vi "PH_IEEE1394Camera.ProcCases.vi"(0 "i ref in":refnum<vi>, 1 "selector":string, 2 "data":T1, 3 "call cluster":T2={"Object"="", "Selector"="", "CallType"=enum."synchronous", "Async Object"="", "Async Selector"="", "Data Descriptor"="", "Data"=[], "Error #"=0, "Expire"=0}, 5 "error in":errorcluster) -> (14 "i ref out":refnum<vi>, 17 "answer cluster":T2={"Object"="", "Selector"="", "CallType"=enum."synchronous", "Async Object"="", "Async Selector"="", "Data Descriptor"="", "Data"=[], "Error #"=0, "Expire"=0}, 19 "error out":errorcluster)   [LabVIEW 2014, in "PH_IEEE1394Camera.lvlib"]
doc: "This method is called by a process from within the default case in the event loop. The methods of a class that are linked to events will be called from THIS method. Add your code here."
uses:
  PH_IEEE1394Camera.lvlib
  CS_Core/CSSystem/CoreDefs/CoreDefs.call_type.ctl
  CS_Core/BaseProcess/BaseProcess.descriptor string definition.ctl
  CS_Core/CSSystem/CoreDefs/CoreDefs.rawDataType.ctl
  CS_Core/CSSystem/CoreLib/CoreLib.string 2 byte array.vi
  CS_Core/CSSystem/CoreLib/CoreLib.byte array 2 int.vi
  CS_Core/CSSystem/CoreLib/CoreLib.byte array 2 double.vi
  CS_Core/CSSystem/CoreLib/CoreLib.byte array 2 short.vi
  CS_Core/CSSystem/CoreLib/CoreLib.byte array 2 string.vi
  CS_Core/CSSystem/CoreLib/CoreLib.lvlib
  CS_Core/BaseProcess/BaseProcess.lvlib
  CS_Core/CAEObj/CAEObj.lvlib
  PH_Basics/PH_PSDBWriter/PH_PSDBWriter.lvlib
  PH_Basics/PH_Cam_BaseClass/PH_Cam_BaseClass.lvlib
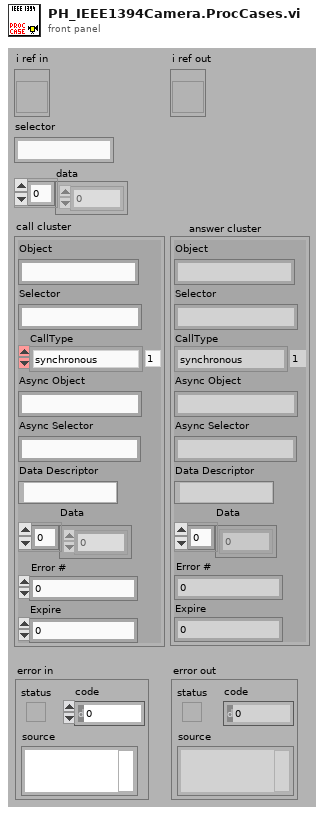
[diagram p1: front panel]
types:
  T1 = typedef "CoreDefs.rawDataType.ctl" = i8[]
  T2 = typedef "CoreDefs.call_type.ctl" = cluster{"Object":string, "Selector":string, "CallType":enum16{"simple", "synchronous", "asynchronous"}, "Async Object":string, "Async Selector":string, "Data Descriptor":T3, "Data":T1, "Error #":i32, "Expire":u32}
  T3 = typedef "BaseProcess.lvlib/BaseProcess.descriptor string definition.ctl" = string
  T4 = typedef "PH_PSDBWriter.lvlib/PH_PSDBWriter.PHELIX-Subsystems.ctl" = i32
  T5 = typedef "PH_IEEE1394Camera.lvlib/PH_IEEE1394Camera.i attribute.ctl" = cluster{"Gui Refs":cluster{"Brightness":refnum<vi>, "Shutter":refnum<vi>, "Gain":refnum<vi>, "Center of Gravity":refnum<vi>, "Supported Video Modes":refnum<vi>, "Trigger Polarity":refnum<vi>, "Trigger Mode":refnum<vi>, "Trigger Timeout":refnum<vi>, "Bit Depth":refnum<vi>, "Video Mode":refnum<vi>, "Top":refnum<vi>, "Bottom":refnum<vi>, "Left":refnum<vi>, "Right":refnum<vi>, "Set ROI to Maximum":refnum<vi>, "Camera Details":refnum<vi>, "Current Cam Attributes":refnum<vi>, "Attribute to set":refnum<vi>, "Num Value":refnum<vi>, "String Value":refnum<vi>, "Bool Value":refnum<vi>, "Set Cam Attribute":refnum<vi>}, "Cam":cluster{"IMAQ1394 Session":T6, "Camera Details":T7}, "Current Attributes":T8[], "Supported Video Modes ":cluster{"Video Mode":u32, "Video Mode Name":string}[], "Wanted Attributes":cluster{"Name":string, "Num Value":dbl, "String Value":string, "Boolean Value":bool}[], "Cam Attributes":T10}
  T6 = typedef "IMAQdx.ctl" = refnum<k21>
  T7 = typedef "PH_IEEE1394Camera.lvlib/PH_IEEE1394Camera.Cam Details.ctl" = cluster{"Model":string, "Serial Number":dbl, "Cam name (Machinery)":string, "Bus Type":string}
  T8 = typedef "PH_IEEE1394Camera.lvlib/PH_IEEE1394Camera.Cam Attribute.ctl" = cluster{"Information":cluster{"Type":T9, "Readable":bool, "Writable":bool, "Name":string}, "Num Value":dbl, "String Value":string, "Maximum":dbl, "Minimum":dbl, "Units":string, "Description":string, "EnumStrings[]":string[], "EnumValues[]":u32[], "Boolean Value":bool}
  T9 = typedef "NI_Vision_Acquisition_Software.lvlib/IMAQdx Attribute Type.ctl" = enum32{"U32", "I64", "DBL", "String", "Enum", "Bool", "Command"}
  T10 = typedef "PH_IEEE1394Camera.lvlib/PH_IEEE1394Camera.Relevant Cam Attributes.ctl" = cluster{"Video Mode":cluster{"Name":string, "Index":i32}, "Brightness":cluster{"Name":string, "Index":i32}, "Gain":cluster{"Name":string, "Index":i32}, "Shutter":cluster{"Name":string, "Index":i32}, "Trigger Pol":cluster{"Name":string, "Index":i32}, "Trigger Mode":cluster{"Name":string, "Index":i32}, "Timeout":cluster{"Name":string, "Index":i32}, "Bit Depth":cluster{"Name":string, "Index":i32}, "Pixel Bits":cluster{"Name":string, "Index":i32}, "Pixel Bytes":cluster{"Name":string, "Index":i32}, "Left":cluster{"Name":string, "Index":i32}, "Right":cluster{"Name":string, "Index":i32}, "Top":cluster{"Name":string, "Index":i32}, "Bottom":cluster{"Name":string, "Index":i32}}
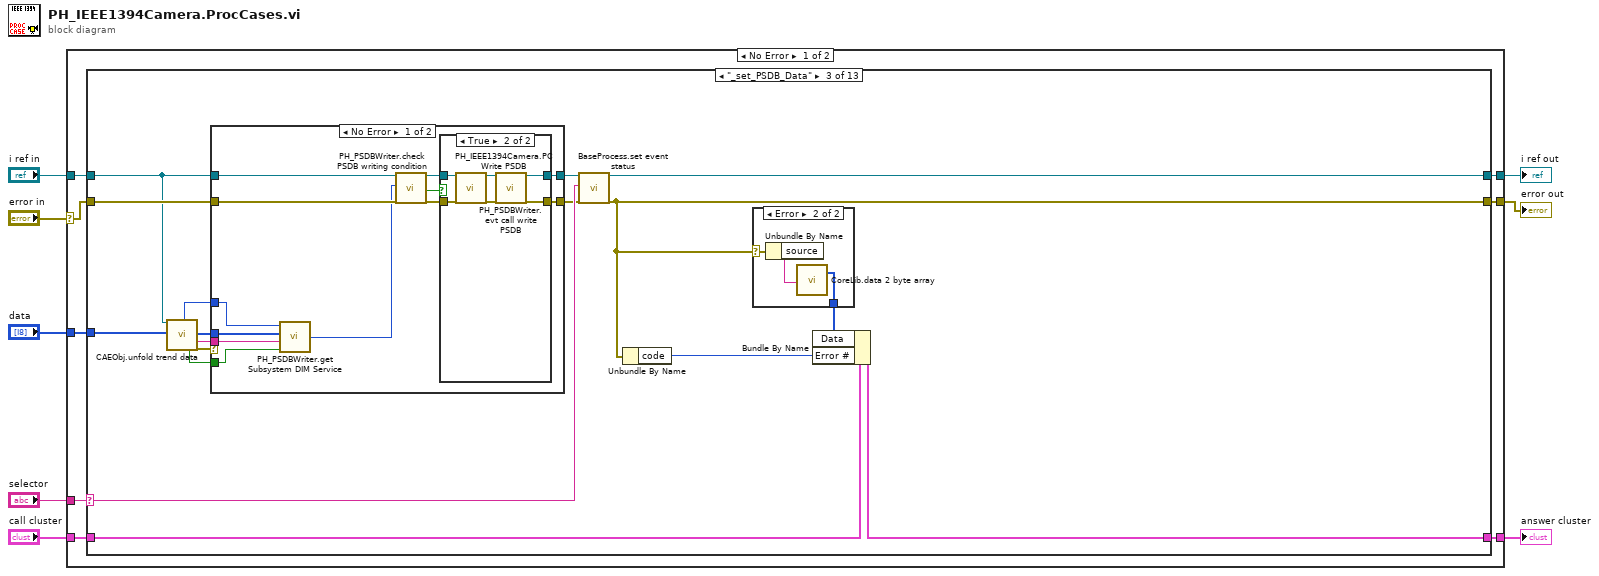
[diagram p0: block diagram]
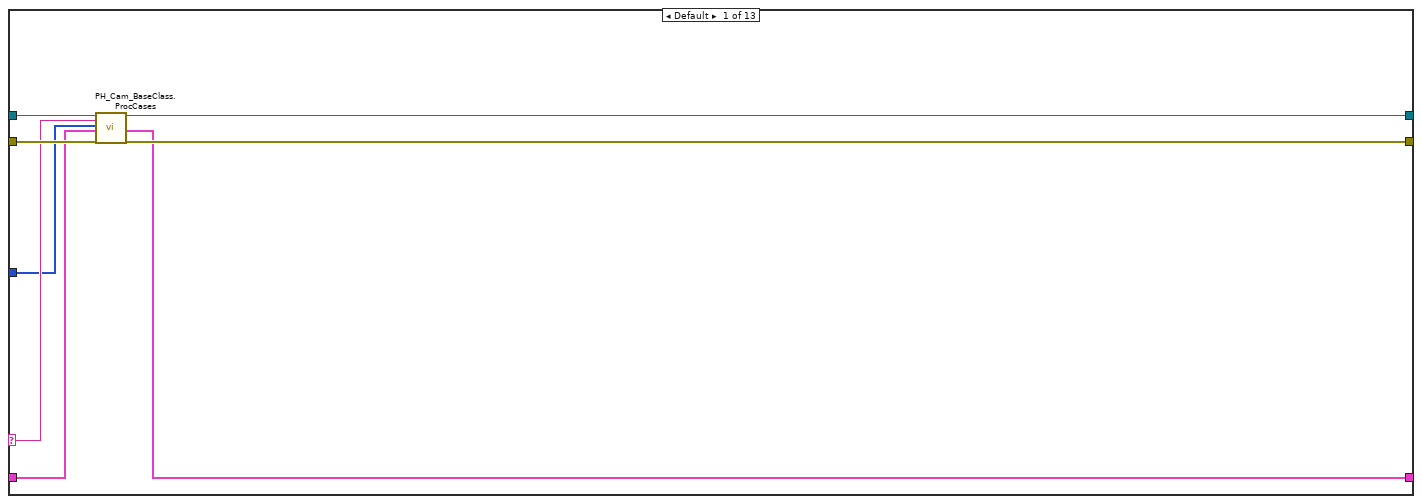
[diagram p2: hidden frame]
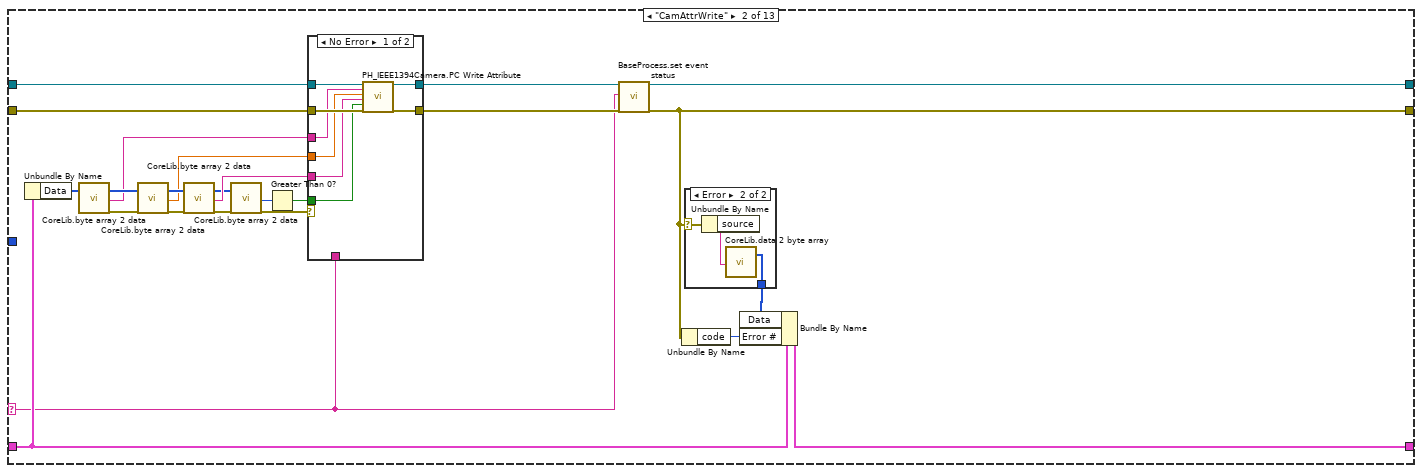
[diagram p3: hidden frame]
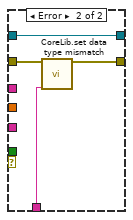
[diagram p5: hidden frame]
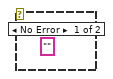
[diagram p8: hidden frame]
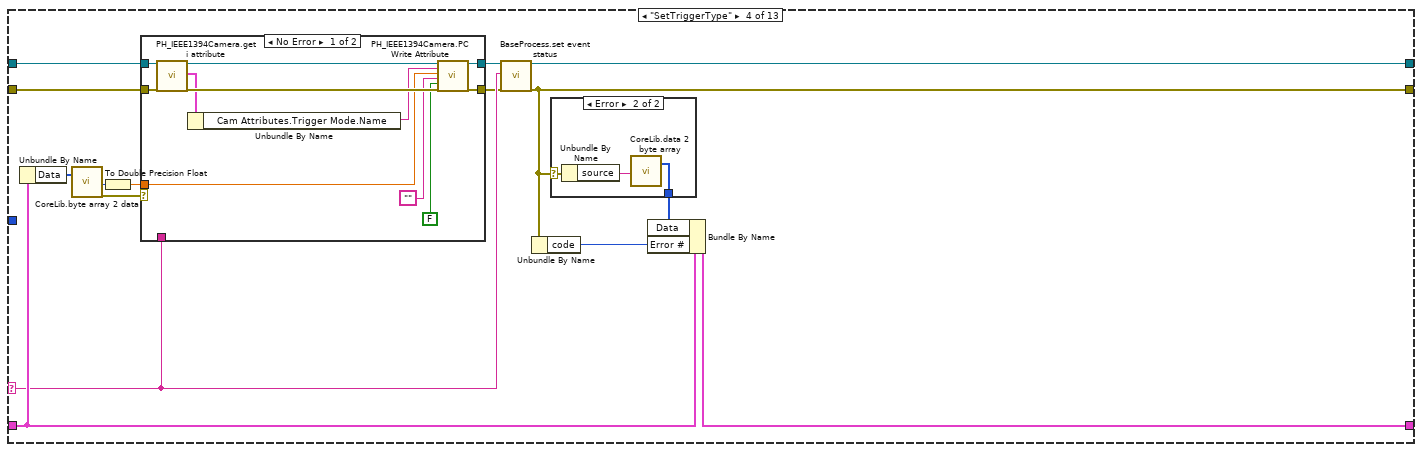
[diagram p9: hidden frame]
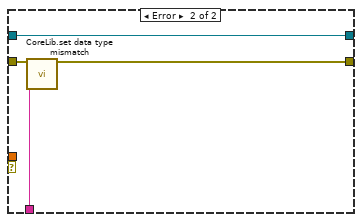
[diagram p10: hidden frame]
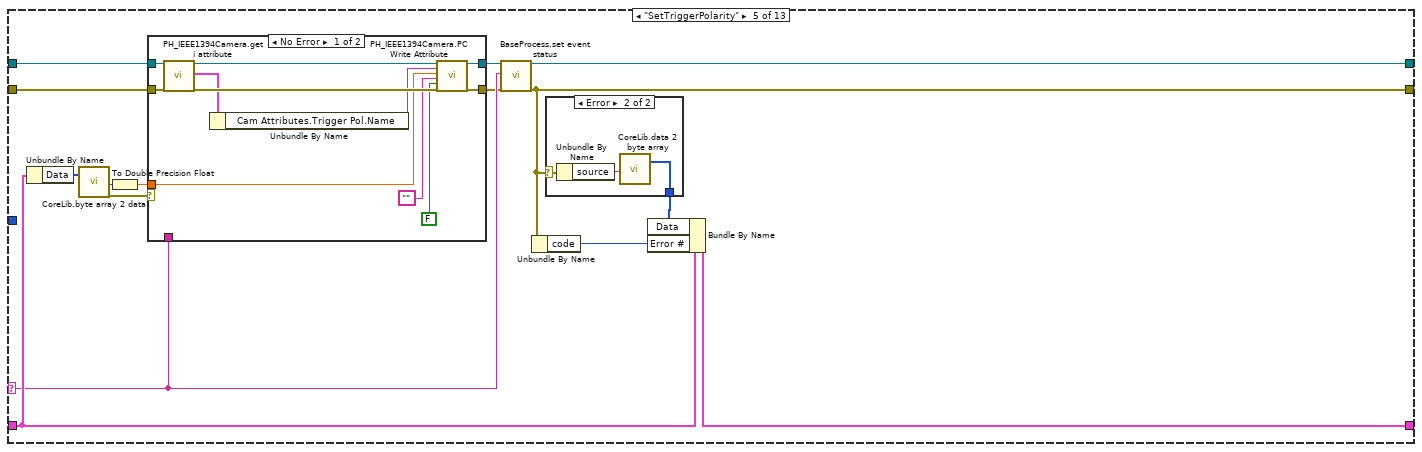
[diagram p12: hidden frame]
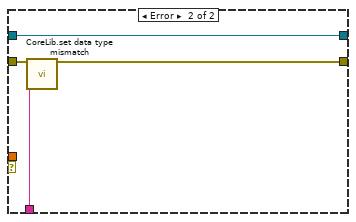
[diagram p13: hidden frame]
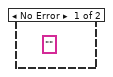
[diagram p14: hidden frame]
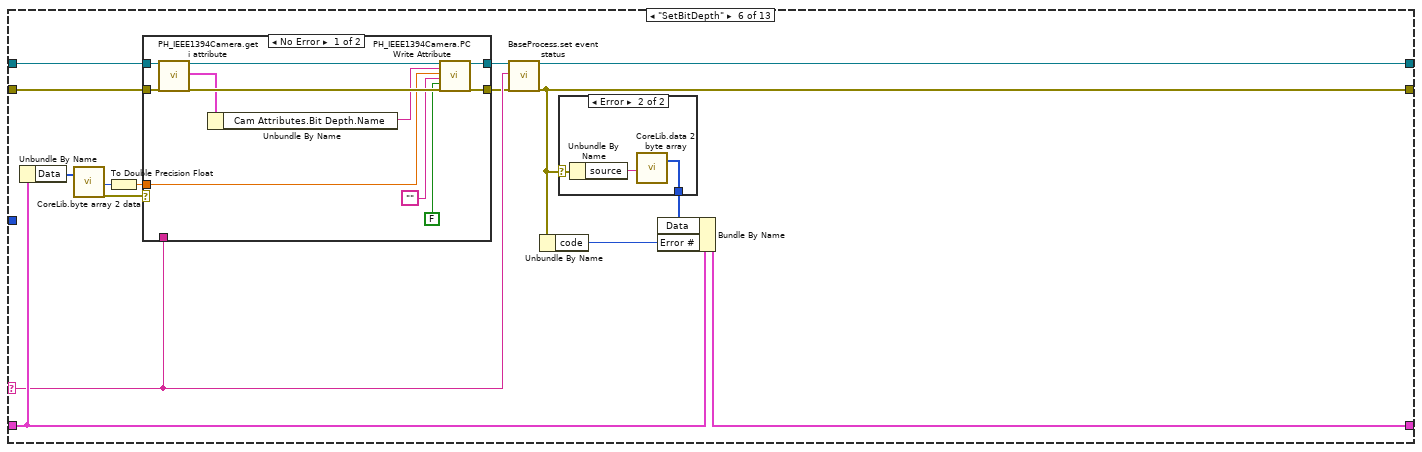
[diagram p15: hidden frame]
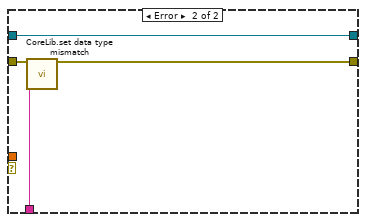
[diagram p16: hidden frame]
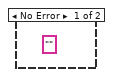
[diagram p17: hidden frame]
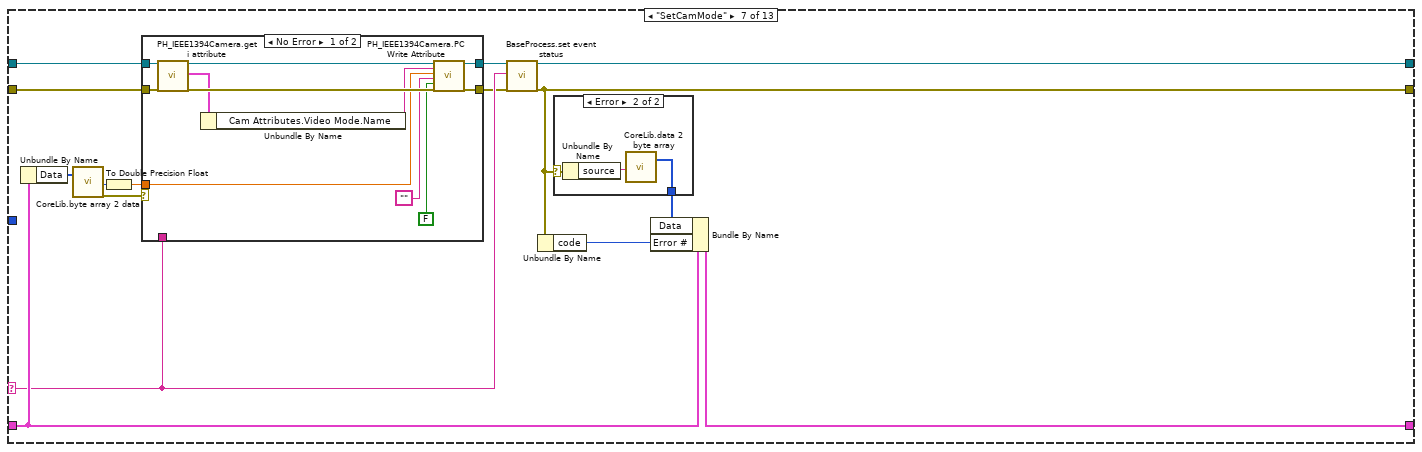
[diagram p18: hidden frame]
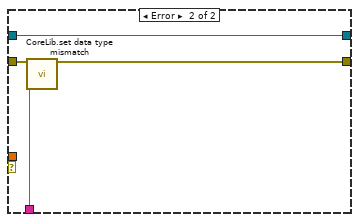
[diagram p19: hidden frame]
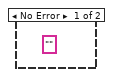
[diagram p20: hidden frame]
diagram:
  n1 = case shown="No Error" "error in" {
    selector: "error in" -> [w9 w553]
    tunnel: "selector" -> [w16 _]
    tunnel: [w15 w552] -> w7
    tunnel: "call cluster" -> [w14 w552]
    tunnel: "i ref in" -> [w13 w554]
    tunnel: [w12 w554] -> w4
    tunnel: [w11 w553] -> w3
    tunnel: "data" -> [w10 _]
    frame No Error {
      n2 = case shown="\"_set_PSDB_Data\"" w16 {
        selector: w16 -> [w19 w40 w76 w111 w141 w175 w207 w241 w273 w305 w336 w381 w501]
        tunnel: w13 -> [w18 w48 w67 w112 w144 w177 w210 w244 w276 w308 w339 w389 w498]
        tunnel: [w24 w39 w75 w116 w150 w182 w216 w248 w280 w312 w345 w380 w500] -> w12
        tunnel: w14 -> [w20 w45 w79 w119 w142 w185 w208 w242 w274 w306 w337 w386 w504]
        tunnel: [w21 w44 w78 w118 w152 w184 w218 w250 w282 w314 w347 w385 w503] -> w15
        tunnel: w9 -> [w23 w47 w68 w110 w143 w176 w209 w243 w275 w307 w338 w388 w497]
        tunnel: [w22 w41 w77 w117 w151 w183 w217 w249 w281 w313 w346 w382 w502] -> w11
        tunnel: w10 -> [w17 _ w64 _ _ _ _ _ _ _ _ _ _]
        frame Default {
          # "In the default case, always call the ProcCase method of the parent class"
          n3 = call "PH_Cam_BaseClass.ProcCases.vi"("i ref in"=w18, "selector"=w19, "data"=w17, "call cluster"=w20, "error in"=w23) -> ("i ref out"=w24:refnum<vi>, "answer cluster"=w21:T2, "error out"=w22:errorcluster)  [unwired: 12 in]
        }
        frame "CamAttrWrite" {
          n4 = Unbundle By Name(w45) -> ("Data"=w28:T1)
          n5 = call-poly "CoreLib.byte array 2 data.vi"("byteArray"=w28) -> ("byteArray out"=w27:T1, "string"=w25:string, "error out"=w26:errorcluster)  [unwired: 16 in]
          n6 = call-poly "CoreLib.byte array 2 data.vi"("byteArray"=w27, "error in (no error)"=w26) -> ("byteArray out"=w36:T1, "d64"=w31:dbl, "error out"=w34:errorcluster)  [unwired: 15 in]
          n7 = call-poly "CoreLib.byte array 2 data.vi"("byteArray"=w36, "error in (no error)"=w34) -> ("byteArray out"=w35:T1, "string"=w37:string, "error out"=w33:errorcluster)  [unwired: 15 in]
          n8 = call-poly "CoreLib.byte array 2 data.vi"("byteArray"=w35, "error in (no error)"=w33) -> ("i16"=w30:i16, "error out"=w32:errorcluster)  [unwired: 15 in, 1 out]
          n9 = Greater Than 0?(x=w30) -> (x > 0?=w29:bool)
          n10 = case shown="No Error" w32 {
            tunnel: [w59 w63] -> w43
            tunnel: w48 -> [w57 w63]
            tunnel: w47 -> [w56 w62]
            tunnel: [w58 w61] -> w42
            tunnel: w40 -> [_ w60]
            tunnel: w37 -> [w54 _]
            tunnel: w31 -> [w53 _]
            tunnel: w29 -> [w55 _]
            tunnel: w25 -> [w52 _]
            frame No Error {
              n11 = call "PH_IEEE1394Camera.PC Write Attribute.vi"("i ref out"=w57, "Attribute Name"=w52, "Wanted Num"=w53, "Wanted String"=w54, "Wanted Bool"=w55, "error out"=w56) -> ("i ref out"=w59:refnum<vi>, "error out"=w58:errorcluster)  [unwired: 12 in]
            }
            frame Error {
              n12 = call "CoreLib.set data type mismatch.vi"("error in (no error)"=w62, "error source"=w60) -> ("error out"=w61:errorcluster)  [unwired: 17 in]
            }
          }
          n13 = call "BaseProcess.set event status.vi"("i ref in"=w43, "EventStatus"=w40, "error in (no error)"=w42) -> ("i ref out"=w39:refnum<vi>, "error out"=w41:errorcluster)  [unwired: 14 in, 1 out]
          n14 = Unbundle By Name(w41) -> ("code"=w46:i32)
          n15 = case shown="Error" w41 {
            selector: w41 -> [_ w51]
            tunnel: [_ w49] -> w38
            frame No Error {
            }
            frame Error {
              n16 = Unbundle By Name(w51) -> ("source"=w50:string)
              n17 = call-poly "CoreLib.data 2 byte array.vi"("string"=w50) -> ("byteArray out"=w49:T1)  [unwired: 18 in]
            }
          }
          n18 = Bundle By Name(cluster=w45, "Data"=w38, "Error #"=w46) -> (w44:T2)
        }
        frame "_set_PSDB_Data" {
          n19 = call "CAEObj.unfold trend data.vi"("i ref in"=w67, "raw trend data"=w64) -> ("quality"=w69:i32, "no link"=w72:bool, "data"=w70:i8[], "typeDescriptor"=w71:string, "error out"=w73:errorcluster)  [unwired: 9 in, 4 out]
          n20 = case shown="No Error" w73 {
            tunnel: w68 -> [w92 w102]
            tunnel: [w91 w101] -> w66
            tunnel: [w90 w102] -> w65
            tunnel: w67 -> [w88 w101]
            tunnel: w72 -> [w82 _]
            tunnel: w71 -> [w84 _]
            tunnel: w70 -> [w85 _]
            tunnel: w69 -> [w83 _]
            frame No Error {
              n21 = call "PH_PSDBWriter.get Subsystem DIM Service.vi"("no link"=w82, "typeDescriptor"=w84, "data"=w85, "quality"=w83) -> ("PHELIX Subsystems"=w81:T4)
              n22 = call "PH_PSDBWriter.check PSDB writing condition.vi"("i ref in"=w88, "wanted Subsystem"=w81, "error IO"=w92) -> ("i ref out"=w87:refnum<vi>, "write PSDB?"=w86:bool, "error out"=w89:errorcluster)  [unwired: 14 in]
              n23 = case shown="True" w86 {
                tunnel: w89 -> [w93 w100]
                tunnel: [w94 w97] -> w91
                tunnel: [w93 w95] -> w90
                tunnel: w87 -> [w94 w99]
                frame False {
                }
                frame True {
                  n24 = call "PH_IEEE1394Camera.PC Write PSDB.vi"("i ref in"=w99, "error IO"=w100) -> ("i ref out"=w98:refnum<vi>, "error out"=w96:errorcluster)  [unwired: 16 in]
                  n25 = call "PH_PSDBWriter.evt call write PSDB.vi"("i ref in"=w98, "error in (no error)"=w96) -> ("i ref out"=w97:refnum<vi>, "error out"=w95:errorcluster)  [unwired: 16 in]
                }
              }
            }
            frame Error {
            }
          }
          n26 = call "BaseProcess.set event status.vi"("i ref in"=w66, "EventStatus"=w76, "error in (no error)"=w65) -> ("i ref out"=w75:refnum<vi>, "error out"=w77:errorcluster)  [unwired: 14 in, 1 out]
          n27 = Unbundle By Name(w77) -> ("code"=w80:i32)
          n28 = case shown="Error" w77 {
            selector: w77 -> [_ w105]
            tunnel: [_ w103] -> w74
            frame No Error {
              (unwired) "" ("source")
            }
            frame Error {
              n29 = Unbundle By Name(w105) -> ("source"=w104:string)
              n30 = call-poly "CoreLib.data 2 byte array.vi"("string"=w104) -> ("byteArray out"=w103:T1)  [unwired: 18 in]
            }
          }
          n31 = Bundle By Name(cluster=w79, "Data"=w74, "Error #"=w80) -> (w78:T2)
        }
        frame "SetTriggerType" {
          n32 = Unbundle By Name(w119) -> ("Data"=w115:T1)
          n33 = call-poly "CoreLib.byte array 2 data.vi"("byteArray"=w115) -> ("i32"=w113:i32, "error out"=w107:errorcluster)  [unwired: 16 in, 1 out]
          n34 = To Double Precision Float(number=w113) -> (double precision float=w106:dbl)
          n35 = case shown="No Error" w107 {
            tunnel: [w126 w135] -> w109
            tunnel: w112 -> [w131 w135]
            tunnel: w110 -> [w130 w134]
            tunnel: [w128 w133] -> w108
            tunnel: w111 -> [_ w132]
            tunnel: w106 -> [w124 _]
            frame No Error {
              n36 = call "PH_IEEE1394Camera.get i attribute.vi"("i ref in"=w131, "error in (no error)"=w130) -> ("i ref out"=w127:refnum<vi>, "i attribute"=w125:T5, "error out"=w129:errorcluster)  [unwired: 15 in]
              n37 = Unbundle By Name(w125) -> ("Cam Attributes.Trigger Mode.Name"=w121:string)
              n38 = call "PH_IEEE1394Camera.PC Write Attribute.vi"("i ref out"=w127, "Attribute Name"=w121, "Wanted Num"=w124, "Wanted String"="", "Wanted Bool"=FALSE, "error out"=w129) -> ("i ref out"=w126:refnum<vi>, "error out"=w128:errorcluster)  [unwired: 12 in]
            }
            frame Error {
              n39 = call "CoreLib.set data type mismatch.vi"("error in (no error)"=w134, "error source"=w132) -> ("error out"=w133:errorcluster)  [unwired: 17 in]
            }
          }
          n40 = call "BaseProcess.set event status.vi"("i ref in"=w109, "EventStatus"=w111, "error in (no error)"=w108) -> ("i ref out"=w116:refnum<vi>, "error out"=w117:errorcluster)  [unwired: 14 in, 1 out]
          n41 = Unbundle By Name(w117) -> ("code"=w120:i32)
          n42 = case shown="Error" w117 {
            selector: w117 -> [_ w138]
            tunnel: [_ w137] -> w114
            frame No Error {
            }
            frame Error {
              n43 = Unbundle By Name(w138) -> ("source"=w136:string)
              n44 = call-poly "CoreLib.data 2 byte array.vi"("string"=w136) -> ("byteArray out"=w137:T1)  [unwired: 18 in]
            }
          }
          n45 = Bundle By Name(cluster=w119, "Data"=w114, "Error #"=w120) -> (w118:T2)
        }
        frame "SetTriggerPolarity" {
          n46 = Unbundle By Name(w142) -> ("Data"=w148:T1)
          n47 = call-poly "CoreLib.byte array 2 data.vi"("byteArray"=w148) -> ("i32"=w147:i32, "error out"=w146:errorcluster)  [unwired: 16 in, 1 out]
          n48 = To Double Precision Float(number=w147) -> (double precision float=w145:dbl)
          n49 = case shown="No Error" w146 {
            tunnel: [w159 w168] -> w140
            tunnel: w144 -> [w164 w168]
            tunnel: w143 -> [w163 w167]
            tunnel: [w161 w166] -> w139
            tunnel: w141 -> [_ w165]
            tunnel: w145 -> [w157 _]
            frame No Error {
              n50 = call "PH_IEEE1394Camera.get i attribute.vi"("i ref in"=w164, "error in (no error)"=w163) -> ("i ref out"=w160:refnum<vi>, "i attribute"=w158:T5, "error out"=w162:errorcluster)  [unwired: 15 in]
              n51 = Unbundle By Name(w158) -> ("Cam Attributes.Trigger Pol.Name"=w154:string)
              n52 = call "PH_IEEE1394Camera.PC Write Attribute.vi"("i ref out"=w160, "Attribute Name"=w154, "Wanted Num"=w157, "Wanted String"="", "Wanted Bool"=FALSE, "error out"=w162) -> ("i ref out"=w159:refnum<vi>, "error out"=w161:errorcluster)  [unwired: 12 in]
            }
            frame Error {
              n53 = call "CoreLib.set data type mismatch.vi"("error in (no error)"=w167, "error source"=w165) -> ("error out"=w166:errorcluster)  [unwired: 17 in]
            }
          }
          n54 = call "BaseProcess.set event status.vi"("i ref in"=w140, "EventStatus"=w141, "error in (no error)"=w139) -> ("i ref out"=w150:refnum<vi>, "error out"=w151:errorcluster)  [unwired: 14 in, 1 out]
          n55 = Unbundle By Name(w151) -> ("code"=w153:i32)
          n56 = case shown="Error" w151 {
            selector: w151 -> [_ w171]
            tunnel: [_ w169] -> w149
            frame No Error {
              (unwired) "" ("source")
            }
            frame Error {
              n57 = Unbundle By Name(w171) -> ("source"=w170:string)
              n58 = call-poly "CoreLib.data 2 byte array.vi"("string"=w170) -> ("byteArray out"=w169:T1)  [unwired: 18 in]
            }
          }
          n59 = Bundle By Name(cluster=w142, "Data"=w149, "Error #"=w153) -> (w152:T2)
        }
        frame "SetBitDepth" {
          n60 = Unbundle By Name(w185) -> ("Data"=w181:T1)
          n61 = call-poly "CoreLib.byte array 2 data.vi"("byteArray"=w181) -> ("i32"=w179:i32, "error out"=w172:errorcluster)  [unwired: 16 in, 1 out]
          n62 = To Double Precision Float(number=w179) -> (double precision float=w178:dbl)
          n63 = case shown="No Error" w172 {
            tunnel: [w192 w201] -> w174
            tunnel: w177 -> [w197 w201]
            tunnel: w176 -> [w196 w200]
            tunnel: [w194 w199] -> w173
            tunnel: w175 -> [_ w198]
            tunnel: w178 -> [w190 _]
            frame No Error {
              n64 = call "PH_IEEE1394Camera.get i attribute.vi"("i ref in"=w197, "error in (no error)"=w196) -> ("i ref out"=w193:refnum<vi>, "i attribute"=w191:T5, "error out"=w195:errorcluster)  [unwired: 15 in]
              n65 = Unbundle By Name(w191) -> ("Cam Attributes.Bit Depth.Name"=w187:string)
              n66 = call "PH_IEEE1394Camera.PC Write Attribute.vi"("i ref out"=w193, "Attribute Name"=w187, "Wanted Num"=w190, "Wanted String"="", "Wanted Bool"=FALSE, "error out"=w195) -> ("i ref out"=w192:refnum<vi>, "error out"=w194:errorcluster)  [unwired: 12 in]
            }
            frame Error {
              n67 = call "CoreLib.set data type mismatch.vi"("error in (no error)"=w200, "error source"=w198) -> ("error out"=w199:errorcluster)  [unwired: 17 in]
            }
          }
          n68 = call "BaseProcess.set event status.vi"("i ref in"=w174, "EventStatus"=w175, "error in (no error)"=w173) -> ("i ref out"=w182:refnum<vi>, "error out"=w183:errorcluster)  [unwired: 14 in, 1 out]
          n69 = Unbundle By Name(w183) -> ("code"=w186:i32)
          n70 = case shown="Error" w183 {
            selector: w183 -> [_ w204]
            tunnel: [_ w203] -> w180
            frame No Error {
              (unwired) "" ("source")
            }
            frame Error {
              n71 = Unbundle By Name(w204) -> ("source"=w202:string)
              n72 = call-poly "CoreLib.data 2 byte array.vi"("string"=w202) -> ("byteArray out"=w203:T1)  [unwired: 18 in]
            }
          }
          n73 = Bundle By Name(cluster=w185, "Data"=w180, "Error #"=w186) -> (w184:T2)
        }
        frame "SetCamMode" {
          n74 = Unbundle By Name(w208) -> ("Data"=w214:T1)
          n75 = call-poly "CoreLib.byte array 2 data.vi"("byteArray"=w214) -> ("i32"=w213:i32, "error out"=w212:errorcluster)  [unwired: 16 in, 1 out]
          n76 = To Double Precision Float(number=w213) -> (double precision float=w211:dbl)
          n77 = case shown="No Error" w212 {
            tunnel: [w225 w234] -> w206
            tunnel: w210 -> [w230 w234]
            tunnel: w209 -> [w229 w233]
            tunnel: [w227 w232] -> w205
            tunnel: w207 -> [_ w231]
            tunnel: w211 -> [w223 _]
            frame No Error {
              n78 = call "PH_IEEE1394Camera.get i attribute.vi"("i ref in"=w230, "error in (no error)"=w229) -> ("i ref out"=w226:refnum<vi>, "i attribute"=w224:T5, "error out"=w228:errorcluster)  [unwired: 15 in]
              n79 = Unbundle By Name(w224) -> ("Cam Attributes.Video Mode.Name"=w220:string)
              n80 = call "PH_IEEE1394Camera.PC Write Attribute.vi"("i ref out"=w226, "Attribute Name"=w220, "Wanted Num"=w223, "Wanted String"="", "Wanted Bool"=FALSE, "error out"=w228) -> ("i ref out"=w225:refnum<vi>, "error out"=w227:errorcluster)  [unwired: 12 in]
            }
            frame Error {
              n81 = call "CoreLib.set data type mismatch.vi"("error in (no error)"=w233, "error source"=w231) -> ("error out"=w232:errorcluster)  [unwired: 17 in]
            }
          }
          n82 = call "BaseProcess.set event status.vi"("i ref in"=w206, "EventStatus"=w207, "error in (no error)"=w205) -> ("i ref out"=w216:refnum<vi>, "error out"=w217:errorcluster)  [unwired: 14 in, 1 out]
          n83 = Unbundle By Name(w217) -> ("code"=w219:i32)
          n84 = case shown="Error" w217 {
            selector: w217 -> [_ w237]
            tunnel: [_ w236] -> w215
            frame No Error {
              (unwired) "" ("source")
            }
            frame Error {
              n85 = Unbundle By Name(w237) -> ("source"=w235:string)
              n86 = call-poly "CoreLib.data 2 byte array.vi"("string"=w235) -> ("byteArray out"=w236:T1)  [unwired: 18 in]
            }
          }
          n87 = Bundle By Name(cluster=w208, "Data"=w215, "Error #"=w219) -> (w218:T2)
        }
        frame "SetBrightness" {
          n88 = Unbundle By Name(w242) -> ("Data"=w246:T1)
          n89 = call-poly "CoreLib.byte array 2 data.vi"("byteArray"=w246) -> ("d64"=w238:dbl, "error out"=w245:errorcluster)  [unwired: 16 in, 1 out]
          n90 = case shown="No Error" w245 {
            tunnel: [w257 w266] -> w239
            tunnel: w244 -> [w262 w266]
            tunnel: w243 -> [w261 w265]
            tunnel: [w259 w264] -> w240
            tunnel: w241 -> [_ w263]
            tunnel: w238 -> [w255 _]
            frame No Error {
              n91 = call "PH_IEEE1394Camera.get i attribute.vi"("i ref in"=w262, "error in (no error)"=w261) -> ("i ref out"=w258:refnum<vi>, "i attribute"=w256:T5, "error out"=w260:errorcluster)  [unwired: 15 in]
              n92 = Unbundle By Name(w256) -> ("Cam Attributes.Brightness.Name"=w252:string)
              n93 = call "PH_IEEE1394Camera.PC Write Attribute.vi"("i ref out"=w258, "Attribute Name"=w252, "Wanted Num"=w255, "Wanted String"="", "Wanted Bool"=FALSE, "error out"=w260) -> ("i ref out"=w257:refnum<vi>, "error out"=w259:errorcluster)  [unwired: 12 in]
            }
            frame Error {
              n94 = call "CoreLib.set data type mismatch.vi"("error in (no error)"=w265, "error source"=w263) -> ("error out"=w264:errorcluster)  [unwired: 17 in]
            }
          }
          n95 = call "BaseProcess.set event status.vi"("i ref in"=w239, "EventStatus"=w241, "error in (no error)"=w240) -> ("i ref out"=w248:refnum<vi>, "error out"=w249:errorcluster)  [unwired: 14 in, 1 out]
          n96 = Unbundle By Name(w249) -> ("code"=w251:i32)
          n97 = case shown="Error" w249 {
            selector: w249 -> [_ w269]
            tunnel: [_ w267] -> w247
            frame No Error {
              (unwired) "" ("source")
            }
            frame Error {
              n98 = Unbundle By Name(w269) -> ("source"=w268:string)
              n99 = call-poly "CoreLib.data 2 byte array.vi"("string"=w268) -> ("byteArray out"=w267:T1)  [unwired: 18 in]
            }
          }
          n100 = Bundle By Name(cluster=w242, "Data"=w247, "Error #"=w251) -> (w250:T2)
        }
        frame "SetShutter" {
          n101 = Unbundle By Name(w274) -> ("Data"=w278:T1)
          n102 = call-poly "CoreLib.byte array 2 data.vi"("byteArray"=w278) -> ("d64"=w270:dbl, "error out"=w277:errorcluster)  [unwired: 16 in, 1 out]
          n103 = case shown="No Error" w277 {
            tunnel: [w289 w298] -> w272
            tunnel: w276 -> [w294 w298]
            tunnel: w275 -> [w293 w297]
            tunnel: [w291 w296] -> w271
            tunnel: w273 -> [_ w295]
            tunnel: w270 -> [w287 _]
            frame No Error {
              n104 = call "PH_IEEE1394Camera.get i attribute.vi"("i ref in"=w294, "error in (no error)"=w293) -> ("i ref out"=w290:refnum<vi>, "i attribute"=w288:T5, "error out"=w292:errorcluster)  [unwired: 15 in]
              n105 = Unbundle By Name(w288) -> ("Cam Attributes.Shutter.Name"=w284:string)
              n106 = call "PH_IEEE1394Camera.PC Write Attribute.vi"("i ref out"=w290, "Attribute Name"=w284, "Wanted Num"=w287, "Wanted String"="", "Wanted Bool"=FALSE, "error out"=w292) -> ("i ref out"=w289:refnum<vi>, "error out"=w291:errorcluster)  [unwired: 12 in]
            }
            frame Error {
              n107 = call "CoreLib.set data type mismatch.vi"("error in (no error)"=w297, "error source"=w295) -> ("error out"=w296:errorcluster)  [unwired: 17 in]
            }
          }
          n108 = call "BaseProcess.set event status.vi"("i ref in"=w272, "EventStatus"=w273, "error in (no error)"=w271) -> ("i ref out"=w280:refnum<vi>, "error out"=w281:errorcluster)  [unwired: 14 in, 1 out]
          n109 = Unbundle By Name(w281) -> ("code"=w283:i32)
          n110 = case shown="Error" w281 {
            selector: w281 -> [_ w301]
            tunnel: [_ w299] -> w279
            frame No Error {
              (unwired) "" ("source")
            }
            frame Error {
              n111 = Unbundle By Name(w301) -> ("source"=w300:string)
              n112 = call-poly "CoreLib.data 2 byte array.vi"("string"=w300) -> ("byteArray out"=w299:T1)  [unwired: 18 in]
            }
          }
          n113 = Bundle By Name(cluster=w274, "Data"=w279, "Error #"=w283) -> (w282:T2)
        }
        frame "SetGain" {
          n114 = Unbundle By Name(w306) -> ("Data"=w310:T1)
          n115 = call-poly "CoreLib.byte array 2 data.vi"("byteArray"=w310) -> ("d64"=w302:dbl, "error out"=w309:errorcluster)  [unwired: 16 in, 1 out]
          n116 = case shown="No Error" w309 {
            tunnel: [w321 w330] -> w304
            tunnel: w308 -> [w326 w330]
            tunnel: w307 -> [w325 w329]
            tunnel: [w323 w328] -> w303
            tunnel: w305 -> [_ w327]
            tunnel: w302 -> [w319 _]
            frame No Error {
              n117 = call "PH_IEEE1394Camera.get i attribute.vi"("i ref in"=w326, "error in (no error)"=w325) -> ("i ref out"=w322:refnum<vi>, "i attribute"=w320:T5, "error out"=w324:errorcluster)  [unwired: 15 in]
              n118 = Unbundle By Name(w320) -> ("Cam Attributes.Gain.Name"=w316:string)
              n119 = call "PH_IEEE1394Camera.PC Write Attribute.vi"("i ref out"=w322, "Attribute Name"=w316, "Wanted Num"=w319, "Wanted String"="", "Wanted Bool"=FALSE, "error out"=w324) -> ("i ref out"=w321:refnum<vi>, "error out"=w323:errorcluster)  [unwired: 12 in]
            }
            frame Error {
              n120 = call "CoreLib.set data type mismatch.vi"("error in (no error)"=w329, "error source"=w327) -> ("error out"=w328:errorcluster)  [unwired: 17 in]
            }
          }
          n121 = call "BaseProcess.set event status.vi"("i ref in"=w304, "EventStatus"=w305, "error in (no error)"=w303) -> ("i ref out"=w312:refnum<vi>, "error out"=w313:errorcluster)  [unwired: 14 in, 1 out]
          n122 = Unbundle By Name(w313) -> ("code"=w315:i32)
          n123 = case shown="Error" w313 {
            selector: w313 -> [_ w333]
            tunnel: [_ w331] -> w311
            frame No Error {
              (unwired) "" ("source")
            }
            frame Error {
              n124 = Unbundle By Name(w333) -> ("source"=w332:string)
              n125 = call-poly "CoreLib.data 2 byte array.vi"("string"=w332) -> ("byteArray out"=w331:T1)  [unwired: 18 in]
            }
          }
          n126 = Bundle By Name(cluster=w306, "Data"=w311, "Error #"=w315) -> (w314:T2)
        }
        frame "SetTimeout" {
          n127 = Unbundle By Name(w337) -> ("Data"=w343:T1)
          n128 = call-poly "CoreLib.byte array 2 data.vi"("byteArray"=w343) -> ("i32"=w342:i32, "error out"=w341:errorcluster)  [unwired: 16 in, 1 out]
          n129 = To Double Precision Float(number=w342) -> (double precision float=w340:dbl)
          n130 = case shown="No Error" w341 {
            tunnel: [w354 w363] -> w334
            tunnel: w339 -> [w359 w363]
            tunnel: w338 -> [w358 w362]
            tunnel: [w356 w361] -> w335
            tunnel: w336 -> [_ w360]
            tunnel: w340 -> [w352 _]
            frame No Error {
              n131 = call "PH_IEEE1394Camera.get i attribute.vi"("i ref in"=w359, "error in (no error)"=w358) -> ("i ref out"=w355:refnum<vi>, "i attribute"=w353:T5, "error out"=w357:errorcluster)  [unwired: 15 in]
              n132 = Unbundle By Name(w353) -> ("Cam Attributes.Timeout.Name"=w349:string)
              n133 = call "PH_IEEE1394Camera.PC Write Attribute.vi"("i ref out"=w355, "Attribute Name"=w349, "Wanted Num"=w352, "Wanted String"="", "Wanted Bool"=FALSE, "error out"=w357) -> ("i ref out"=w354:refnum<vi>, "error out"=w356:errorcluster)  [unwired: 12 in]
            }
            frame Error {
              n134 = call "CoreLib.set data type mismatch.vi"("error in (no error)"=w362, "error source"=w360) -> ("error out"=w361:errorcluster)  [unwired: 17 in]
            }
          }
          n135 = call "BaseProcess.set event status.vi"("i ref in"=w334, "EventStatus"=w336, "error in (no error)"=w335) -> ("i ref out"=w345:refnum<vi>, "error out"=w346:errorcluster)  [unwired: 14 in, 1 out]
          n136 = Unbundle By Name(w346) -> ("code"=w348:i32)
          n137 = case shown="Error" w346 {
            selector: w346 -> [_ w366]
            tunnel: [_ w364] -> w344
            frame No Error {
              (unwired) "" ("source")
            }
            frame Error {
              n138 = Unbundle By Name(w366) -> ("source"=w365:string)
              n139 = call-poly "CoreLib.data 2 byte array.vi"("string"=w365) -> ("byteArray out"=w364:T1)  [unwired: 18 in]
            }
          }
          n140 = Bundle By Name(cluster=w337, "Data"=w344, "Error #"=w348) -> (w347:T2)
        }
        frame "SetROI" {
          n141 = Unbundle By Name(w386) -> ("Data"=w379:T1)
          n142 = call-poly "CoreLib.byte array 2 data.vi"("byteArray"=w379) -> ("byteArray out"=w372:T1, "i32"=w378:i32, "error out"=w374:errorcluster)  [unwired: 16 in]
          n143 = call-poly "CoreLib.byte array 2 data.vi"("byteArray"=w372, "error in (no error)"=w374) -> ("byteArray out"=w371:T1, "i32"=w369:i32, "error out"=w376:errorcluster)  [unwired: 15 in]
          n144 = call-poly "CoreLib.byte array 2 data.vi"("byteArray"=w371, "error in (no error)"=w376) -> ("byteArray out"=w370:T1, "i32"=w368:i32, "error out"=w375:errorcluster)  [unwired: 15 in]
          n145 = call-poly "CoreLib.byte array 2 data.vi"("byteArray"=w370, "error in (no error)"=w375) -> ("i32"=w367:i32, "error out"=w373:errorcluster)  [unwired: 15 in, 1 out]
          n146 = case shown="No Error" w373 {
            tunnel: [w412 w479] -> w384
            tunnel: w389 -> [w404 w479]
            tunnel: w388 -> [w403 w478]
            tunnel: [w411 w477] -> w383
            tunnel: w381 -> [_ w476]
            tunnel: w378 -> [w420 _]
            tunnel: w369 -> [w419 _]
            tunnel: w368 -> [w418 _]
            tunnel: w367 -> [w417 _]
            frame No Error {
              n147 = call "PH_IEEE1394Camera.get i attribute.vi"("i ref in"=w404, "error in (no error)"=w403) -> ("i ref out"=w402:refnum<vi>, "i attribute"=w405:T5, "error out"=w401:errorcluster)  [unwired: 15 in]
              n148 = Unbundle By Name(w405) -> ("Cam Attributes"=w395:T10, "Cam Attributes.Bottom.Index"=w406:i32, "Cam Attributes.Top.Index"=w407:i32, "Cam Attributes.Right.Index"=w408:i32, "Cam Attributes.Left.Index"=w409:i32, "Current Attributes"=w410:T8[])
              n149 = To Unsigned Long Integer(number=w420) -> (unsigned 32bit integer=w416:u32)
              n150 = To Unsigned Long Integer(number=w419) -> (unsigned 32bit integer=w415:u32)
              n151 = To Unsigned Long Integer(number=w418) -> (unsigned 32bit integer=w414:u32)
              n152 = To Unsigned Long Integer(number=w417) -> (unsigned 32bit integer=w413:u32)
              n153 = Build Array(w406, w407, w408, w409) -> (w399:i32[])
              n154 = Not Equal?(x=w399, y=-1) -> (x != y?=w397:bool[])
              n155 = And Array Elements(Boolean array=w397) -> (logical AND=w396:bool)
              n156 = case shown="True" w396 {
                tunnel: w416 -> [w431 w453]
                tunnel: w415 -> [w430 w452]
                tunnel: w414 -> [w429 w451]
                tunnel: w413 -> [w428 w450]
                tunnel: [w427 w432] -> w393
                tunnel: w399 -> [_ w439]
                tunnel: w410 -> [_ w438]
                tunnel: [w421 w437] -> w400
                tunnel: w395 -> [w426 _]
                frame False {
                  n157 = Unbundle By Name(w426) -> ("Top.Name"=w425:string, "Bottom.Name"=w424:string, "Left.Name"=w423:string, "Right.Name"=w422:string)
                  n158 = Build Array(w425, w424, w423, w422) -> (w421:string[])
                  n159 = Build Array(w431, w430, w429, w428) -> (w427:u32[])
                }
                frame True {
                  n160 = for {
                    tunnel: w438 -> [w463]
                    tunnel: w439 -> [w454] mode=indexing
                    tunnel: [w458] -> w440 mode=indexing
                    tunnel: [w457] -> w445 mode=indexing
                    tunnel: [w455] -> w437 mode=indexing
                    n161 = for {
                      tunnel: w463 -> [w467] mode=indexing
                      tunnel: [w466] -> w462 mode=indexing
                      tunnel: [w465] -> w459 mode=indexing
                      tunnel: [w464] -> w456 mode=indexing
                      n162 = Unbundle By Name(w467) -> ("Information.Name"=w464:string, "Maximum"=w466:dbl, "Minimum"=w465:dbl)
                    }
                    n163 = To Unsigned Long Integer(number=w462) -> (unsigned 32bit integer=w461:u32[])
                    n164 = To Unsigned Long Integer(number=w459) -> (unsigned 32bit integer=w460:u32[])
                    n165 = Index Array(array=w456, index=w454) -> (element=w455:string)
                    n166 = Index Array(array=w461, index=w454) -> (element=w458:u32)
                    n167 = Index Array(array=w460, index=w454) -> (element=w457:u32)
                  }
                  n168 = Index Array(array=w440, index #1=0 ("index"), index #2=2 ("index")) -> (element #1=w435:u32, element #2=w433:u32)
                  n169 = Index Array(array=w445, index #1=1 ("index"), index #2=3 ("index")) -> (element #1=w434:u32, element #2=w436:u32)
                  n170 = call "PH_IEEE1394Camera.set ROI Pair.vi"("Lower Limit"=w434, "Input 2"=w452, "Input 1"=w453, "Upper Limit"=w435) -> ("Lower Output"=w448:u32, "Higher Output"=w449:u32)
                  n171 = call "PH_IEEE1394Camera.set ROI Pair.vi"("Lower Limit"=w436, "Input 2"=w450, "Input 1"=w451, "Upper Limit"=w433) -> ("Lower Output"=w446:u32, "Higher Output"=w447:u32)
                  n172 = Build Array(w449, w448, w447, w446) -> (w432:u32[])
                }
              }
              n173 = To Double Precision Float(number=w393) -> (double precision float=w394:dbl[])
              n174 = for {
                shift-right: [w474] -> w412
                shift-left: w402 -> [w475]
                shift-right: [w473] -> w411
                shift-left: w401 -> [w472]
                tunnel: w394 -> [w471] mode=indexing
                tunnel: w400 -> [w468] mode=indexing
                n175 = call "PH_IEEE1394Camera.PC Write Attribute.vi"("i ref out"=w475, "Attribute Name"=w468, "Wanted Num"=w471, "Wanted String"="", "Wanted Bool"=FALSE, "error out"=w472) -> ("i ref out"=w474:refnum<vi>, "error out"=w473:errorcluster)  [unwired: 12 in]
              }
            }
            frame Error {
              n176 = call "CoreLib.set data type mismatch.vi"("error in (no error)"=w478, "error source"=w476) -> ("error out"=w477:errorcluster)  [unwired: 17 in]
            }
          }
          n177 = call "BaseProcess.set event status.vi"("i ref in"=w384, "EventStatus"=w381, "error in (no error)"=w383) -> ("i ref out"=w380:refnum<vi>, "error out"=w382:errorcluster)  [unwired: 14 in, 1 out]
          n178 = Unbundle By Name(w382) -> ("code"=w387:i32)
          n179 = case shown="Error" w382 {
            selector: w382 -> [_ w392]
            tunnel: [_ w390] -> w377
            frame No Error {
              (unwired) "" ("source")
            }
            frame Error {
              n180 = Unbundle By Name(w392) -> ("source"=w391:string)
              n181 = call-poly "CoreLib.data 2 byte array.vi"("string"=w391) -> ("byteArray out"=w390:T1)  [unwired: 18 in]
            }
          }
          n182 = Bundle By Name(cluster=w386, "Data"=w377, "Error #"=w387) -> (w385:T2)
        }
        frame "SetROIMAX" {
          n183 = call "PH_IEEE1394Camera.get i attribute.vi"("i ref in"=w498, "error in (no error)"=w497) -> ("i ref out"=w488:refnum<vi>, "i attribute"=w489:T5, "error out"=w487:errorcluster)  [unwired: 15 in]
          n184 = Unbundle By Name(w489) -> ("Cam Attributes"=w480:T10, "Cam Attributes.Bottom.Index"=w490:i32, "Cam Attributes.Top.Index"=w491:i32, "Cam Attributes.Right.Index"=w492:i32, "Cam Attributes.Left.Index"=w493:i32, "Current Attributes"=w494:T8[])
          n185 = Build Array(w490, w491, w492, w493) -> (w483:i32[])
          n186 = Not Equal?(x=w483, y=-1) -> (x != y?=w482:bool[])
          n187 = And Array Elements(Boolean array=w482) -> (logical AND=w481:bool)
          n188 = case shown="True" w481 {
            tunnel: w494 -> [_ w522]
            tunnel: [w509 w521] -> w486
            tunnel: [w508 w518] -> w485
            tunnel: w483 -> [_ w515]
            tunnel: w480 -> [w514 _]
            frame False {
              w506 = 10000.0 ("element")
              w507 = 0.0 ("element")
              n189 = Unbundle By Name(w514) -> ("Left.Name"=w513:string, "Right.Name"=w512:string, "Top.Name"=w511:string, "Bottom.Name"=w510:string)
              n190 = Build Array(w513, w512, w511, w510) -> (w509:string[])
              n191 = Build Array(w507, w506, w507, w506) -> (w508:dbl[])
            }
            frame True {
              n192 = for {
                tunnel: w522 -> [w536]
                tunnel: w515 -> [w529] mode=indexing
                tunnel: [w535] -> w523 mode=indexing
                tunnel: [w534] -> w528 mode=indexing
                tunnel: [w531] -> w521 mode=indexing
                n193 = for {
                  tunnel: w536 -> [w540] mode=indexing
                  tunnel: [w539] -> w533 mode=indexing
                  tunnel: [w538] -> w532 mode=indexing
                  tunnel: [w537] -> w530 mode=indexing
                  n194 = Unbundle By Name(w540) -> ("Information.Name"=w537:string, "Maximum"=w539:dbl, "Minimum"=w538:dbl)
                }
                n195 = Index Array(array=w530, index=w529) -> (element=w531:string)
                n196 = Index Array(array=w533, index=w529) -> (element=w535:dbl)
                n197 = Index Array(array=w532, index=w529) -> (element=w534:dbl)
              }
              n198 = Index Array(array=w523, index #1=0 ("index"), index #2=2 ("index")) -> (element #1=w520:dbl, element #2=w517:dbl)
              n199 = Index Array(array=w528, index #1=1 ("index"), index #2=3 ("index")) -> (element #1=w516:dbl, element #2=w519:dbl)
              n200 = Build Array(w520, w516, w517, w519) -> (w518:dbl[])
            }
          }
          n201 = for {
            shift-right: [w547] -> w496
            shift-left: w488 -> [w548]
            shift-right: [w546] -> w495
            shift-left: w487 -> [w545]
            tunnel: w485 -> [w544] mode=indexing
            tunnel: w486 -> [w541] mode=indexing
            n202 = call "PH_IEEE1394Camera.PC Write Attribute.vi"("i ref out"=w548, "Attribute Name"=w541, "Wanted Num"=w544, "Wanted String"="", "Wanted Bool"=FALSE, "error out"=w545) -> ("i ref out"=w547:refnum<vi>, "error out"=w546:errorcluster)  [unwired: 12 in]
          }
          n203 = call "BaseProcess.set event status.vi"("i ref in"=w496, "EventStatus"=w501, "error in (no error)"=w495) -> ("i ref out"=w500:refnum<vi>, "error out"=w502:errorcluster)  [unwired: 14 in, 1 out]
          n204 = Unbundle By Name(w502) -> ("code"=w505:i32)
          n205 = case shown="Error" w502 {
            selector: w502 -> [_ w551]
            tunnel: [_ w549] -> w499
            frame No Error {
              (unwired) "" ("source")
            }
            frame Error {
              n206 = Unbundle By Name(w551) -> ("source"=w550:string)
              n207 = call-poly "CoreLib.data 2 byte array.vi"("string"=w550) -> ("byteArray out"=w549:T1)  [unwired: 18 in]
            }
          }
          n208 = Bundle By Name(cluster=w504, "Data"=w499, "Error #"=w505) -> (w503:T2)
        }
      }
    }
    frame Error {
    }
  }
  "answer cluster" <- w7
  "i ref out" <- w4
  "error out" <- w3
